vi "fftGetMagsPoly.vi"   [LabVIEW 2011]
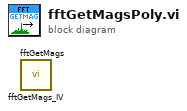
[diagram p0: block diagram]
diagram:
  n1 = call "fftGetMags_IV.vi"() -> ()  [unwired: 12 in, 4 out]
  n2 = call "fftGetMags.vi"() -> ()  [unwired: 13 in, 3 out]
